vi "niRFUtil WFM Apply IQ Perturbations.vi"(0 "Complex Signal In":T2 {"y" format="%.2f"; "dx" format="%^.2e"; "x0" format="%^.2e"}, 5 "I/Q Perturbations":T1={"Mode"=enum."Disabled", "Gain Imbalance (dB)"=0.0, "Quadrature Skew (deg)"=0.0, "I Offset (%)"=0.0, "Q Offset (%)"=0.0, "Frequency Offset (Hz)"=0.0, "Eb/No or SNR (dB)"=inf} {"Eb/No or SNR (dB)" format="%.2f"; "Frequency Offset (Hz)" format="%^.3e"; "Q Offset (%)" format="%.2f"; "I Offset (%)" format="%.2f"; "Quadrature Skew (deg)" format="%.2f"; "Gain Imbalance (dB)" format="%.2f"}, 7 "SPS":i32=16, 9 "Bits/Symbol":i32=1, 11 "error in (no error)":errorcluster) -> (4 "Complex Signal Out":T2 {"y" format="%.2f"; "dx" format="%^.2e"; "x0" format="%^.2e"}, 15 "error out":errorcluster)   [LabVIEW 2015, in "niRFUtil.lvlib"]
doc: "(c) Copyright 2006, National Instruments, Inc. This VI may not be duplicated, sold, or distributed without written consent from National Instruments."
uses:
  niRFUtil.lvlib
  Includes/niRFUtil INC Complex Waveform.ctl
  Includes/niRFUtil INC Complex Array.ctl
  Includes/niRFUtil INC IQ Perturbations.ctl
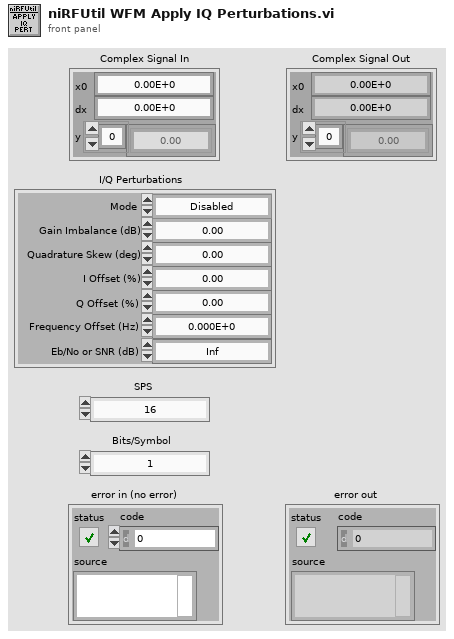
[diagram p1: front panel]
types:
  T1 = typedef "niRFUtil.lvlib/niRFUtil INC IQ Perturbations.ctl" = cluster{"Mode":enum16{"Disabled", "Enabled"}, "Gain Imbalance (dB)":dbl, "Quadrature Skew (deg)":dbl, "I Offset (%)":dbl, "Q Offset (%)":dbl, "Frequency Offset (Hz)":dbl, "Eb/No or SNR (dB)":dbl}
  T2 = typedef "niRFUtil.lvlib/niRFUtil INC Complex Waveform.ctl" = cluster{"x0":dbl, "dx":dbl, "y":T3}
  T3 = typedef "niRFUtil.lvlib/niRFUtil INC Complex Array.ctl" = csg[]
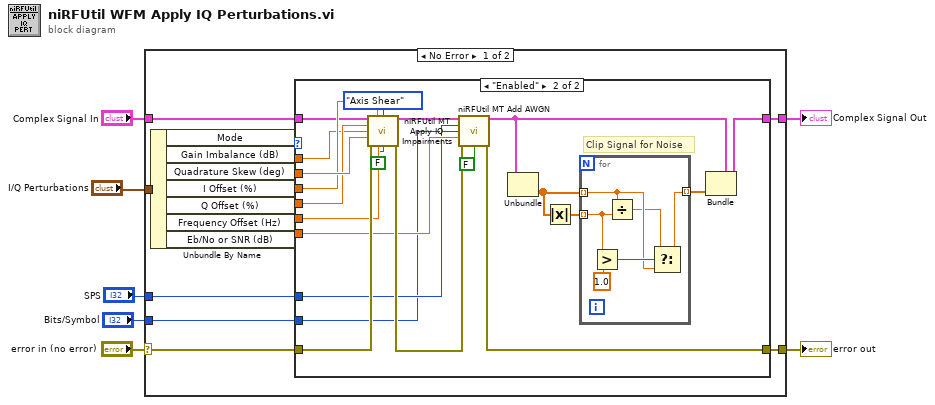
[diagram p0: block diagram]
diagram:
  n1 = case shown="No Error" "error in (no error)" {
    selector: "error in (no error)" -> [w21 w51]
    tunnel: "Complex Signal In" -> [w11 _]
    tunnel: [w20 w51] -> w7
    tunnel: "I/Q Perturbations" -> [w19 _]
    tunnel: [w8 _] -> w1
    tunnel: "SPS" -> [w10 _]
    tunnel: "Bits/Symbol" -> [w9 _]
    frame No Error {
      n2 = Unbundle By Name(w19) -> ("Mode"=w18:enum16{"Disabled", "Enabled"}, "Gain Imbalance (dB)"=w13:dbl, "Quadrature Skew (deg)"=w17:dbl, "I Offset (%)"=w16:dbl, "Q Offset (%)"=w15:dbl, "Frequency Offset (Hz)"=w14:dbl, "Eb/No or SNR (dB)"=w12:dbl)
      n3 = case shown="\"Enabled\"" w18 {
        tunnel: w21 -> [w23 w43]
        tunnel: [w23 w41] -> w20
        tunnel: w17 -> [_ w40]
        tunnel: w16 -> [_ w39]
        tunnel: w15 -> [_ w38]
        tunnel: w14 -> [_ w37]
        tunnel: w13 -> [_ w36]
        tunnel: w12 -> [_ w35]
        tunnel: w11 -> [w22 w30]
        tunnel: [w22 w25] -> w8
        tunnel: w10 -> [_ w32]
        tunnel: w9 -> [_ w31]
        frame "Disabled", Default {
        }
        frame "Enabled" {
          # "Clip Signal for Noise"
          n4 = call "niRFUtil MT Apply IQ Impairments.vi"("Waveform In"=w30, "I DC offset (%)"=w39, "impairment definition"=enum16{"Vertical Shear", "Axis Shear"}."Axis Shear", "Q DC offset (%)"=w38, "IQ gain imbalance (dB)"=w36, "quadrature skew (deg)"=w40, "error in (no error)"=w43, "frequency offset (Hz)"=w37, "reset? (T)"=FALSE) -> ("Waveform Out"=w44:T2, "error out"=w42:errorcluster)  [unwired: 5 in]
          n5 = call "niRFUtil MT Add AWGN.vi"("Waveform In"=w44, "samples per symbol (16)"=w32, "bits per symbol (1)"=w31, "Eb/N0 (10 dB)"=w35, "error in (no error)"=w42, "reset? (T)"=FALSE) -> ("Waveform Out"=w27:T2, "error out"=w41:errorcluster)  [unwired: 7 in, 1 out]
          n6 = Unbundle(w27) -> ("y"=w28:T3)  [unwired: 2 out]
          n7 = Absolute Value(x=w28) -> (abs(x)=w29:sgl[])
          n8 = for {
            tunnel: w29 -> [w48] mode=indexing
            tunnel: w28 -> [w47] mode=indexing
            tunnel: [w45] -> w26 mode=indexing
            n9 = Greater?(x=w48, y=1.0) -> (0:w49:bool)
            n10 = Divide(x=w47, y=w48) -> (x/y=w46:csg)
            n11 = Select(t=w46, s=w49, f=w47) -> (s? t:f=w45:csg)
          }
          n12 = Bundle(cluster=w27, "y"=w26) -> (w25:T2)  [unwired: 2 out]
        }
      }
    }
    frame Error {
    }
  }
  "error out" <- w7
  "Complex Signal Out" <- w1
